vi "E14_FormulaGeneral.vi"() -> ()   [LabVIEW 2026]
panel:
  out "XY Graph":cluster{dbl[], dbl[]}(graph)
  out "Estado de raiz":string
  out "X2":string
  out "X1":string
  in  "Calcular":bool
  in  "c":dbl
  in  "b":dbl
  in  "a":dbl
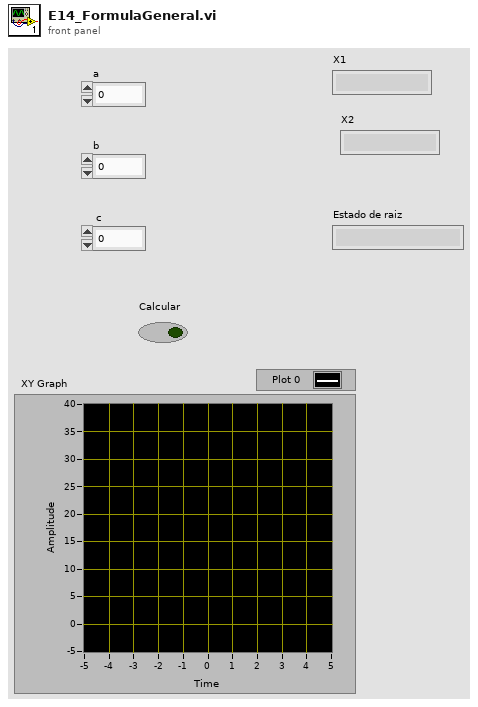
[diagram p1: front panel]
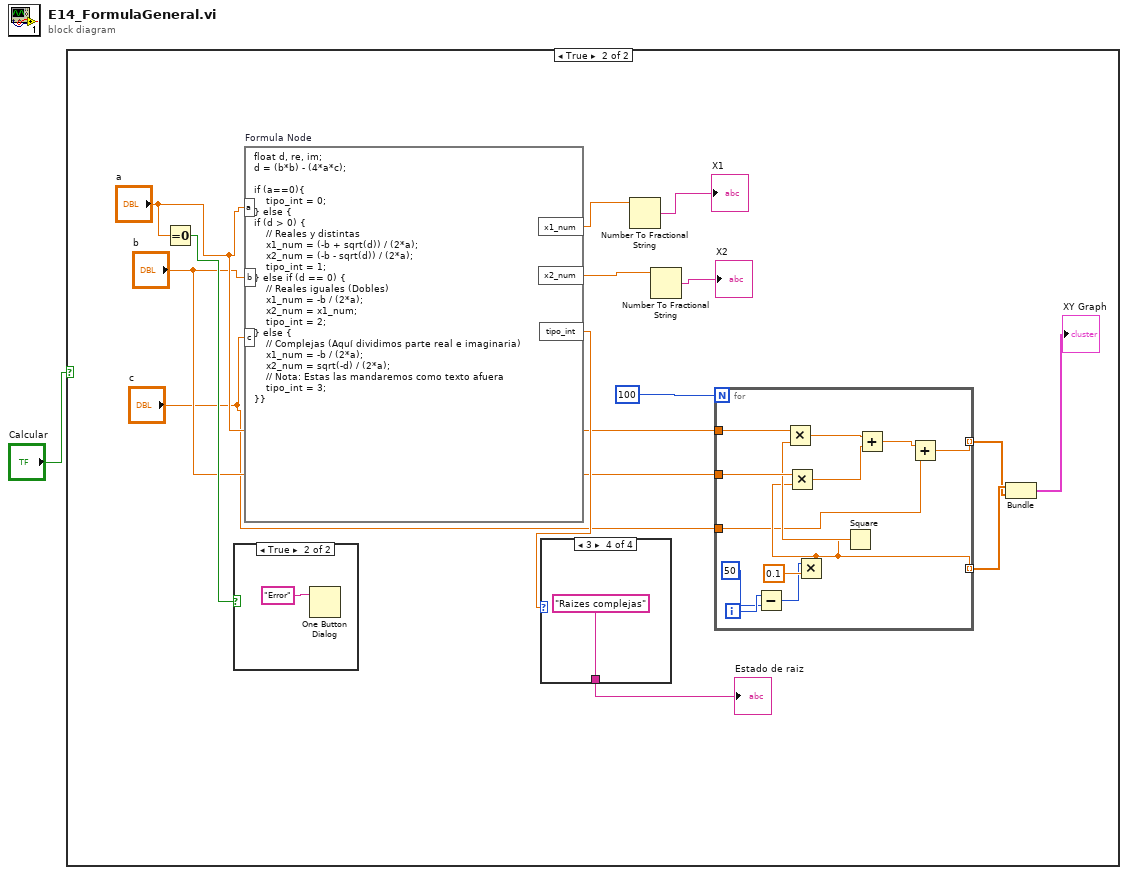
[diagram p0: block diagram]
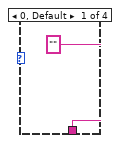
[diagram p4: hidden frame]
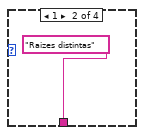
[diagram p5: hidden frame]
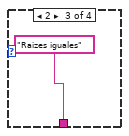
[diagram p6: hidden frame]
diagram:
  n1 = case shown="True" "Calcular" {
    frame False {
    }
    frame True {
      n2 = Equal To 0?(x="a") -> (x = 0?=w10:bool)
      n3 = case shown="True" w10 {
        frame False {
        }
        frame True {
          n4 = One Button Dialog(message="Error") -> ()  [unwired: 1 in, 1 out]
        }
      }
      n5 = formula code="float d, re, im;\nd = (b*b) - (4*a*c);\n\nif (a==0){\n    tipo_int = 0;\n} else {\nif (d > 0) {\n    // Reales y distintas\n    x1_num = (-b + sqrt(d)) / (2*a);\n    x2_num = (-b - sqrt(d)) / (2*a);\n    tipo_int = 1; \n} else if (d == 0) {\n    // Reales iguales (Dobles)\n    x1_num = -b / (2*a);\n    x2_num = x1_num;\n    tipo_int = 2;\n} else {\n    // Complejas (Aquí dividimos parte real e imaginaria)\n    x1_num = -b / (2*a);\n    x2_num = sqrt(-d) / (2*a);\n    // Nota: Estas las mandaremos como texto afuera\n    tipo_int = 3;\n}}"("a"="a", "b"="b", "c"="c") -> ("x1_num"=w13:dbl, "x2_num"=w12:dbl, "tipo_int"=w11:dbl)
      n6 = case shown="3" w11 {
        tunnel: ["" "Raizes distintas" "Raizes iguales" "Raizes complejas"] -> w9
        frame 0, Default {
        }
        frame 1 {
        }
        frame 2 {
        }
        frame 3 {
        }
      }
      "Estado de raiz" <- w9
      n7 = Number To Fractional String(number=w13) -> (F-format string=→"X1":string)  [unwired: 3 in]
      n8 = Number To Fractional String(number=w12) -> (F-format string=→"X2":string)  [unwired: 3 in]
      n9 = for {
        N: 100 -> [_]
        tunnel: [w21] -> w7 mode=indexing
        tunnel: [w16] -> w5 mode=indexing
        tunnel: "a" -> [w24]
        tunnel: "b" -> [w23]
        tunnel: "c" -> [w19]
        i -> [w28]
        n10 = Subtract(x=w28, y=50 ("x")) -> (x-y=w25:i32)
        n11 = Multiply(x=w25, y=0.1) -> (x*y=w21:dbl)
        n12 = Multiply(x=w23, y=w21) -> (x*y=w18:dbl)
        n13 = Square(x=w21) -> (x^2=w22:dbl)
        n14 = Multiply(x=w24, y=w22) -> (x*y=w20:dbl)
        n15 = Add(x=w20, y=w18) -> (x+y=w17:dbl)
        n16 = Add(x=w17, y=w19) -> (x+y=w16:dbl)
      }
      n17 = Bundle "Bundle"(w7, w5) -> (→"XY Graph":cluster{dbl[], dbl[]})  [unwired: 1 in]
    }
  }
